vi "ReceiveNorification.vi"(8 "error in (no error)":errorcluster, 11 "StatisticsDisplay in":refnum<class "Log Notification to File.lvclass">) -> (0 "error out":errorcluster, 3 "StatisticsDisplay out":refnum<class "Log Notification to File.lvclass">)   [LabVIEW 2020, in "Log Notification to File.lvclass"]
uses:
  Log Notification to File.lvclass
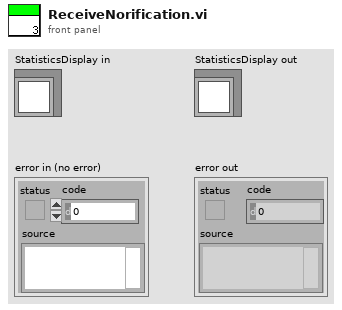
[diagram p1: front panel]
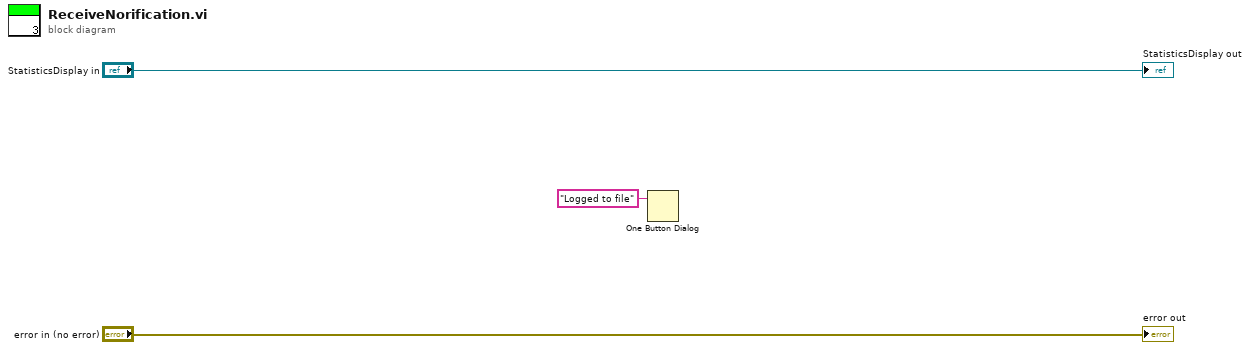
[diagram p0: block diagram]
diagram:
  n1 = One Button Dialog(message="Logged to file") -> ()  [unwired: 1 in, 1 out]
  "error out" <- "error in (no error)"
  "StatisticsDisplay out" <- "StatisticsDisplay in"
